vi "数组字符串加码-数组至字符串.vi"(0 "数组":string[](array[string]), 1 "分隔字符":string="#") -> (2 "字符串":string="123123\\21312\\123123")   [LabVIEW 2014]
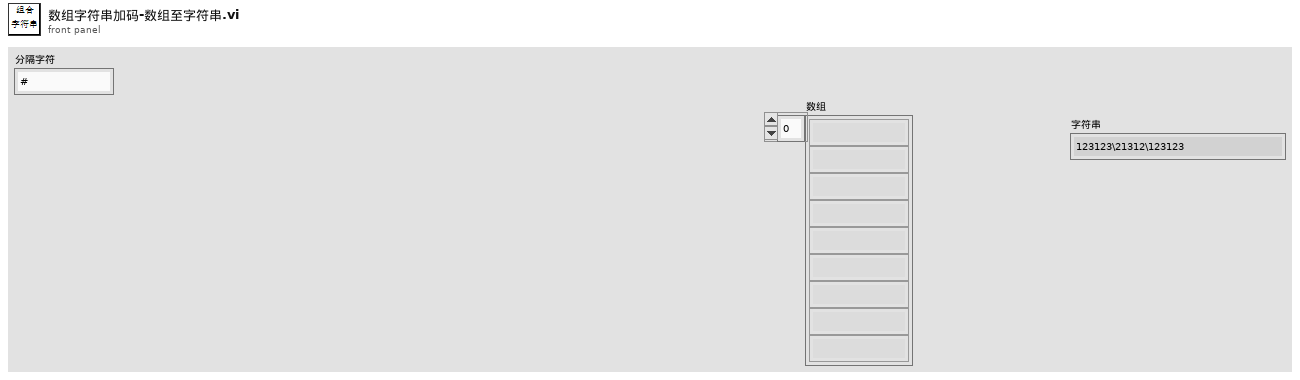
[diagram p1: front panel]
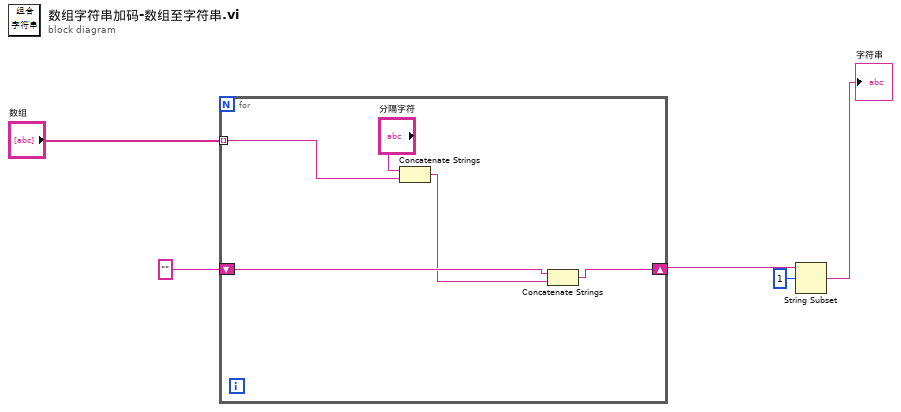
[diagram p0: block diagram]
diagram:
  n1 = for {
    tunnel: "数组" -> [w10] mode=indexing
    shift-right: [w6] -> w3
    shift-left: "" -> [w8]
    n2 = Concatenate Strings("分隔字符", w10) -> (w7:string)
    n3 = Concatenate Strings(w8, w7) -> (w6:string)
  }
  n4 = String Subset(string=w3, offset (0)=1 ("偏移量(0)")) -> (substring=→"字符串":string)  [unwired: 1 in]
